vi "mks670_enable_average.vi"() -> ()   [LabVIEW 2019]
panel:
  out "Command Read":string
  out "tpg361_visa 3":refnum<visa-resource-name>
  out "err_out 2":errorcluster
  out "Status":bool
  in  "tpg361_b2r":u32
  in  "err_in":errorcluster
  in  "tpg361_delay":u32=500
  in  "tpg361_visa":refnum<visa-resource-name>
  # "VISA"
  # "DELAY"
  # "BYTE AT PORT"
  # "STATUS"
  # "ERROR"
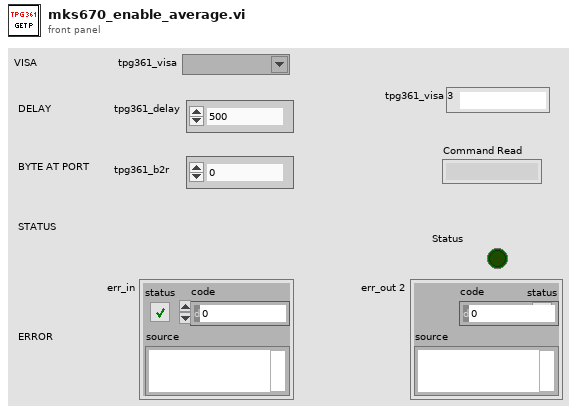
[diagram p1: front panel]
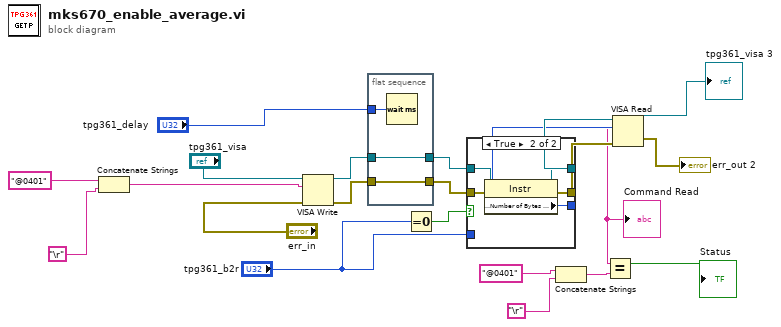
[diagram p0: block diagram]
diagram:
  n1 = Concatenate Strings("@0401" ("string"), "\r") -> (w10:string)
  n2 = VISA Write(VISA resource name="tpg361_visa", write buffer=w10, error in (no error)="err_in") -> (VISA resource name out=w20:refnum<visa-resource-name>, error out=w22:errorcluster)  [unwired: 1 out]
  n3 = flat-sequence {
    tunnel: w22 -> [w24]
    tunnel: [w24] -> w21
    tunnel: w20 -> [w23]
    tunnel: [w23] -> w19
    tunnel: "tpg361_delay" -> [w25]
    frame #0 {
      n4 = Wait (ms)(milliseconds to wait=w25) -> ()  [unwired: 1 out]
    }
  }
  n5 = Equal To 0?(x="tpg361_b2r") -> (x = 0?=w15:bool)
  n6 = case shown="True" w15 {
    tunnel: w21 -> [w27 w33]
    tunnel: w19 -> [w28 w32]
    tunnel: [w28 w31] -> w13
    tunnel: [w27 w30] -> w12
    tunnel: [w26 w29] -> w11
    tunnel: "tpg361_b2r" -> [w26 _]
    frame False {
    }
    frame True {
      n7 = property class="Instr"(reference=w32, error in=w33) -> (reference out=w31:refnum<visa-resource-name>, error out=w30:errorcluster, "Serial Settings:Number of Bytes at Serial Port"=w29:u32)
    }
  }
  n8 = Concatenate Strings("@0401" ("y"), "\r") -> (w1:string)
  n9 = VISA Read(VISA resource name=w13, byte count=w11, error in (no error)=w12) -> (VISA resource name out=→"tpg361_visa 3":refnum<visa-resource-name>, read buffer=w8:string, error out=→"err_out 2":errorcluster)  [unwired: 1 out]
  "Command Read" <- w8
  n10 = Equal?(x=w8, y=w1) -> (x = y?=→"Status":bool)
